vi "Report Core.vi"(8 "error in":errorcluster, 9 "Received":path, 10 "Approved":path, 11 "Report With Custom DiffTool in":refnum<class "Report With Custom DiffTool.lvclass">) -> (0 "error out":errorcluster, 2 "Worked?":bool, 3 "Report With Custom DiffTool out":refnum<class "Report With Custom DiffTool.lvclass">)   [LabVIEW 2020, in "Approval Tests.lvlib" / "Report With Custom DiffTool.lvclass"]
uses:
  Report With Custom DiffTool.lvclass
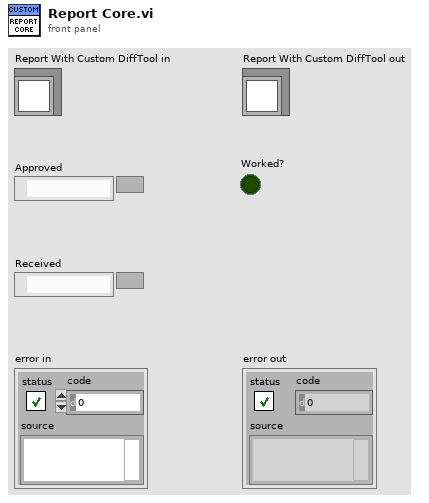
[diagram p1: front panel]
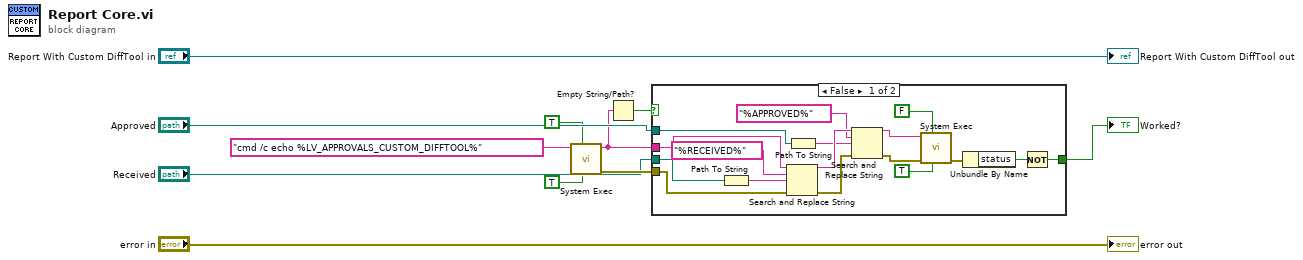
[diagram p0: block diagram]
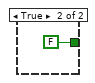
[diagram p2: hidden frame]
diagram:
  n1 = call <vilib>:"System Exec.vi"("run minimized? (F)"=TRUE, "wait until completion? (T)"=TRUE, "command line"="cmd /c echo %LV_APPROVALS_CUSTOM_DIFFTOOL%") -> ("error out"=w10:errorcluster, "standard output"=w2:string)  [unwired: 5 in, 2 out]
  n2 = Empty String/Path?(string/path=w2) -> (empty?=w1:bool)
  n3 = case shown="False" w1 {
    tunnel: "Received" -> [w17 _]
    tunnel: "Approved" -> [w16 _]
    tunnel: [w13 FALSE] -> w6
    tunnel: w10 -> [w26 _]
    tunnel: w2 -> [w12 _]
    frame False {
      n4 = Path To String(path=w17) -> (string=w14:string)
      n5 = Search and Replace String(input string=w12, search string="%RECEIVED%", replace string=w14, error in=w26) -> (result string=w20:string, error out=w27:errorcluster)  [unwired: 4 in, 2 out]
      n6 = Path To String(path=w16) -> (string=w15:string)
      n7 = Search and Replace String(input string=w20, search string="%APPROVED%", replace string=w15, error in=w27) -> (result string=w21:string, error out=w25:errorcluster)  [unwired: 4 in, 2 out]
      n8 = call <vilib>:"System Exec.vi"("run minimized? (F)"=TRUE, "wait until completion? (T)"=FALSE, "error in (no error)"=w25, "command line"=w21) -> ("error out"=w28:errorcluster)  [unwired: 4 in, 3 out]
      n9 = Unbundle By Name(w28) -> ("status"=w23:bool)
      n10 = Not(x=w23) -> (.not. x?=w13:bool)
    }
    frame True {
    }
  }
  "Worked?" <- w6
  "error out" <- "error in"
  "Report With Custom DiffTool out" <- "Report With Custom DiffTool in"
